vi "Class to Variant.vi"(8 "error in (no error)":errorcluster, 10 "Data in":variant, 11 "VI Analyzer Node in":refnum<class "VI Tester Node.lvclass">) -> (0 "error out":errorcluster, 1 "Serialized Object Name":string, 2 "Data Out":variant, 3 "VI Analyzer Node out":refnum<class "VI Tester Node.lvclass">)   [LabVIEW 2014, in "VI Tester Node.lvclass"]
uses:
  VI Tester Node.lvclass
  Shared/Controls/VI Tester - STYP.ctl
  VI Tester Node.lvclass/VI Tester Node.ctl
  Classes/Build Job/Build Job.lvclass
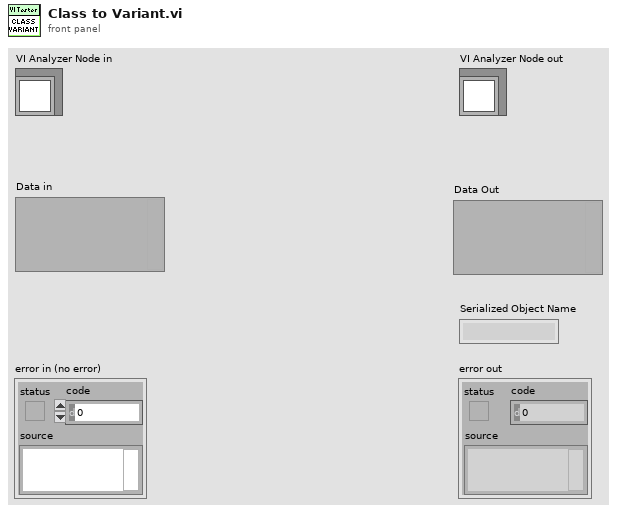
[diagram p1: front panel]
types:
  T1 = typedef "VI Tester - STYP.ctl" = cluster{"Executor_Number":string, "Workspace_Path":string, "Test Case":string}
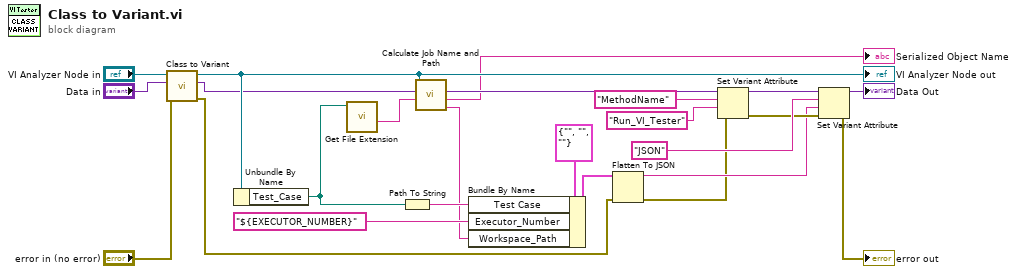
[diagram p0: block diagram]
diagram:
  n1 = call-parent "Class to Variant.vi"("error in (no error)"="error in (no error)", "Data in"="Data in", "Build Job in"="VI Analyzer Node in") -> ("error out"=w3:errorcluster, "Data Out"=w4:variant, "Build Job out"=w18:refnum<class "VI Tester Node.lvclass">)  [unwired: 5 in, 1 out]
  "VI Analyzer Node out" <- w18
  n2 = Unbundle By Name(w18) -> ("Test_Case"=w19:path)
  n3 = call <vilib>:"Get File Extension.vi"("file"=w19) -> ("filename without extension"=w2:string)  [unwired: 7 in, 3 out]
  n4 = Path To String(path=w19) -> (string=w21:string)
  n5 = call "Calculate Job Name and Path.vi"("Job Target"=w2, "Data in"=w4, "Build Job"=w18) -> ("Workspace Path"=w1:string, "Job Name"=→"Serialized Object Name":string, "Data out"=w10:variant)  [unwired: 6 in]
  n6 = Bundle By Name(cluster=T1 {"Executor_Number"="", "Workspace_Path"="", "Test Case"=""} ("VI Tester - STYP.ctl"), "Test Case"=w21, "Executor_Number"="${EXECUTOR_NUMBER}", "Workspace_Path"=w1) -> (w7:T1)
  n7 = Flatten To JSON(anything=w7, error in (no error)=w3) -> (JSON string=w11:string, 11:w8:errorcluster)  [unwired: 1 in]
  n8 = Set Variant Attribute(Variant=w10, name="MethodName", value="Run_VI_Tester", error in=w8) -> (Variant out=w14:variant, error out=w12:errorcluster)  [unwired: 1 out]
  n9 = Set Variant Attribute(Variant=w14, name="JSON" ("Name"), value=w11, error in=w12) -> (Variant out=→"Data Out":variant, error out=→"error out":errorcluster)  [unwired: 1 out]
